vi "Create Custom Error.vi"(3 "show call chain? (T)":bool=TRUE, 5 "enable (T)":bool=TRUE, 7 "code (5000)":i32=5000, 10 "error in":errorcluster, 11 "error message":string) -> (2 "error out":errorcluster)   [LabVIEW 2020, in "g-sugar.lvlib"]
doc: "Generate a new custom error. Use the <b>enable</b> input for conditional errors."
uses:
  g-sugar.lvlib
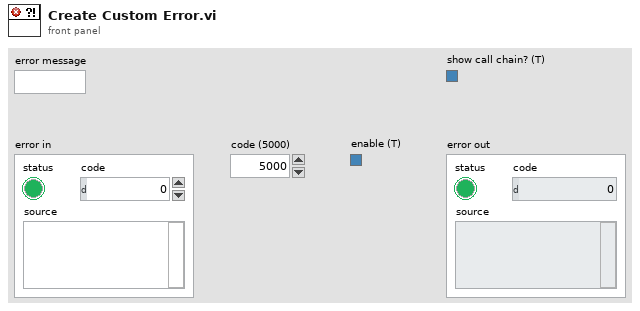
[diagram p1: front panel]
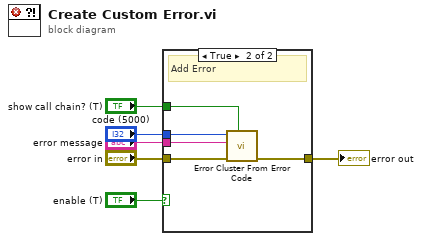
[diagram p0: block diagram]
diagram:
  n1 = case shown="True" "enable (T)" {
    tunnel: "code (5000)" -> [_ w12]
    tunnel: "show call chain? (T)" -> [_ w11]
    tunnel: "error message" -> [_ w10]
    tunnel: "error in" -> [w7 w9]
    tunnel: [w7 w8] -> w2
    frame False {
      # "Don't Add Error"
    }
    frame True {
      # "Add Error"
      n2 = call <vilib>:"Error Cluster From Error Code.vi"("show call chain? (False)"=w11, "error in (no error)"=w9, "error message (\"\")"=w10, "error code (0)"=w12) -> ("error out"=w8:errorcluster)  [unwired: 5 in]
    }
  }
  "error out" <- w2
